vi "CONEX-PP-example.vi"(8 "error in (no error)":errorcluster, 9 "Input Value":string, 10 "Enum":T1(ring), 11 "VISA resource name":refnum<visa-resource-name>="COM6") -> (0 "error out read":errorcluster, 2 "Position":dbl)   [LabVIEW 2020]
doc: "This example performs a serial port write and a serial port read. The parameters set for the serial port must match the parameters of the connected instrument or device. The VISA Configure Serial Port VI sets the configuration parameters. The front panel displays the controls used to configure the basic parameters, such as baud rate, data bits, and parity. The VI passes the VISA resource name to other VIs that perform operations on that VISA resource. The VISA Write function sends a command to the serial device and the VISA Read function returns data based on the command. The VISA Close function then closes the reference to the serial device. It is important to close the reference; otherwise, further communication through that port might not be possible."
uses:
  Serial - Settings.ctl
panel:
  out "Velocity":dbl
  out "Acceleration":dbl
  out "error out write":errorcluster
  out "String 2":string
  in  "Serial Settings":T2={"baud rate"=115200, "data bits"=8, "parity"=enum."None", "stop bits"=10, "flow control"=0} {"flow control" items=["None"=0, "XON/XOFF"=1, "RTS/CTS"=2, "DTR/DSR"=4]; "stop bits" items=["1.0"=10, "1.5"=15, "2.0"=20]; "data bits" min=5 max=8 step=1; "baud rate" items=["75"=75, "110"=110, "134"=134, "150"=150, "300"=300, "600"=600, "1200"=1200, "1800"=1800, "2400"=2400, "4800"=4800, "7200"=7200, "9600"=9600, "14400"=14400, "19200"=19200, "28800"=28800, "38400"=38400, "56000"=56000, "57600"=57600, "115200"=115200, "128000"=128000, "230400"=230400]}
  out "bytes read":u32
  in  "delay before read (ms)":u32=500
  out "Response":string
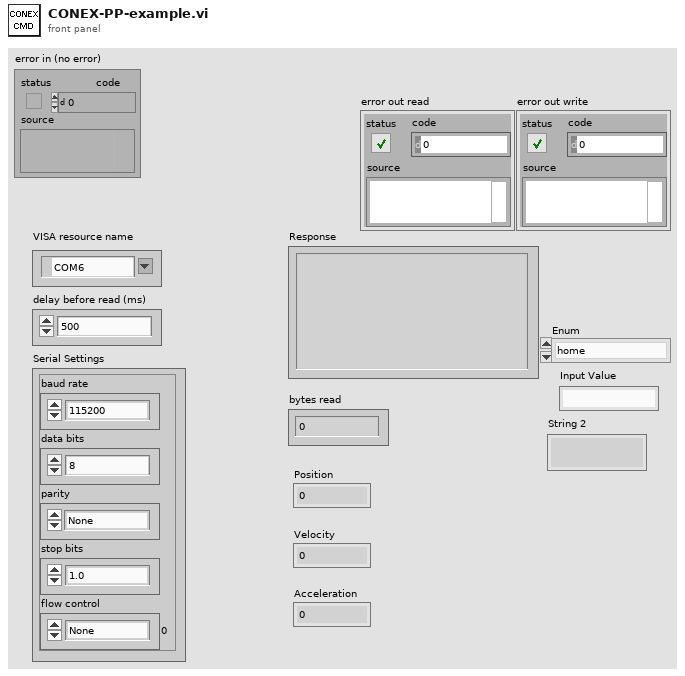
[diagram p1: front panel]
types:
  T1 = enum16{"home", "set position", "get position", "set velocity", "get velocity", "set acceleration", "get acceleration", "abort move", "get configuration", "reset controller", "custom command"}
  T2 = typedef "Serial - Settings.ctl" = cluster{"baud rate":u32, "data bits":u16, "parity":enum16{"None", "Odd", "Even", "Mark", "Space"}, "stop bits":u16, "flow control":u16}
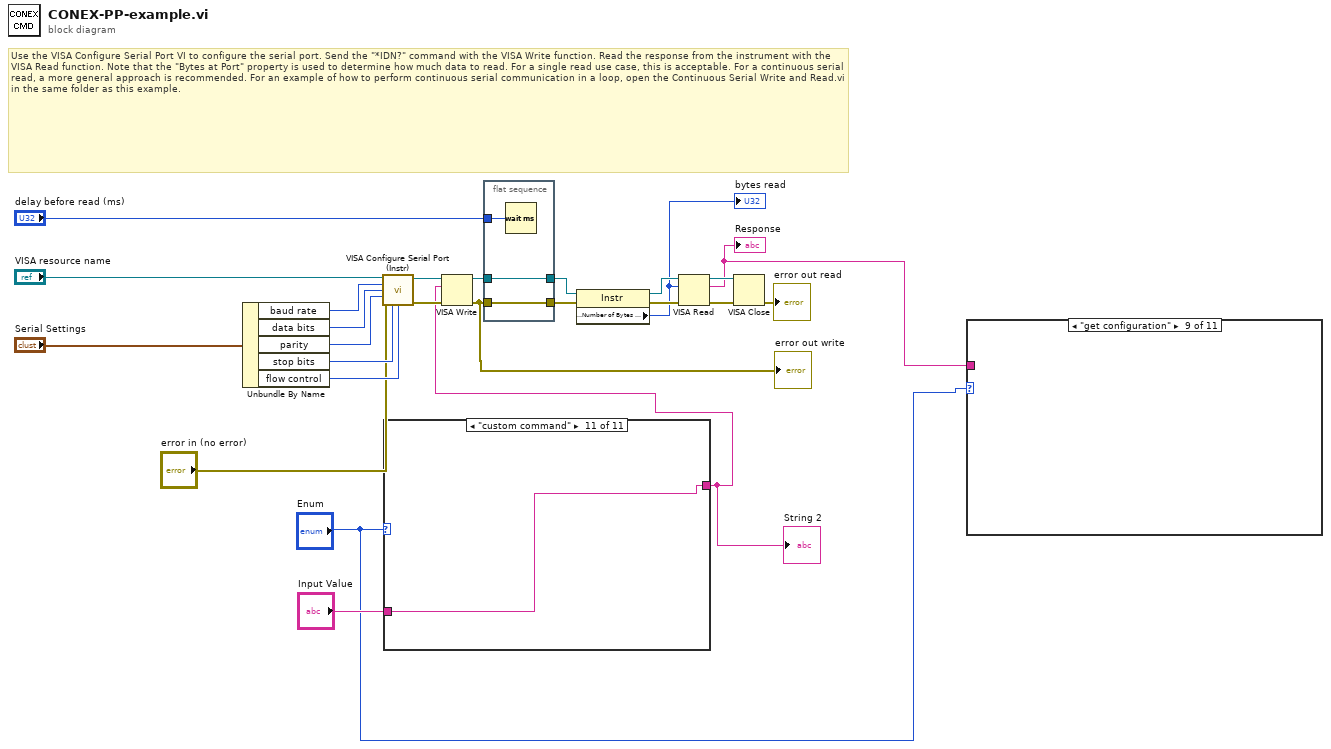
[diagram p0: block diagram]
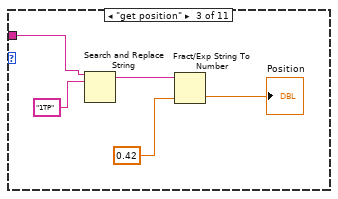
[diagram p4: hidden frame]
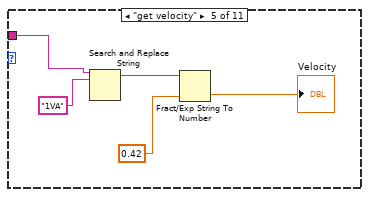
[diagram p6: hidden frame]
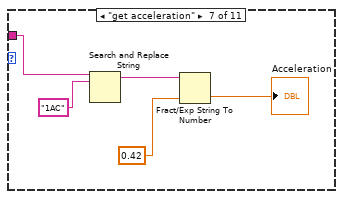
[diagram p8: hidden frame]
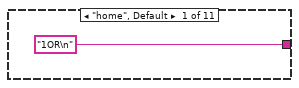
[diagram p12: hidden frame]
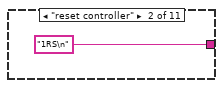
[diagram p13: hidden frame]
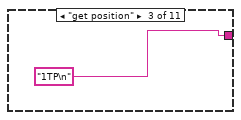
[diagram p14: hidden frame]
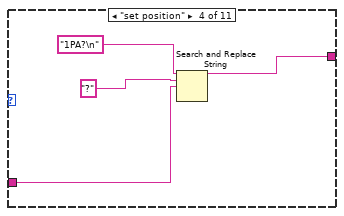
[diagram p15: hidden frame]
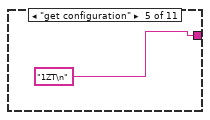
[diagram p16: hidden frame]
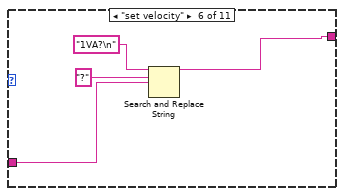
[diagram p17: hidden frame]
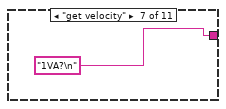
[diagram p18: hidden frame]
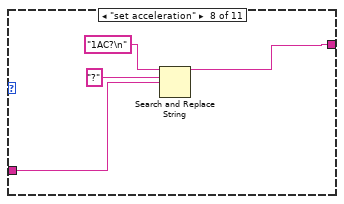
[diagram p19: hidden frame]
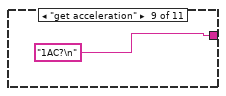
[diagram p20: hidden frame]
diagram:
  # "Use the VISA Configure Serial Port VI to configure the serial port. Send the \"*IDN?\" command with the VISA Write function. Read the response from the instrument with the VISA Read function. Note that the \"Bytes at Port\" property is used to determine how much data to read. For a single read use case, this is acceptable. For a continuous serial read, a more general approach is recommended. For an example of how to perform continuous serial communication in a loop, open the Continuous Serial Write and Read.vi in the same folder as this example."
  n1 = Unbundle By Name("Serial Settings") -> ("baud rate"=w12:u32, "data bits"=w11:u16, "parity"=w10:enum16{"None", "Odd", "Even", "Mark", "Space"}, "stop bits"=w9:u16, "flow control"=w8:u16)
  n2 = call "VISA Configure Serial Port (Instr).vi"("VISA resource name"="VISA resource name", "baud rate (9600)"=w12, "data bits (8)"=w11, "parity (0:none)"=w10, "error in (no error)"="error in (no error)", "stop bits (10: 1 bit)"=w9, "flow control (0:none)"=w8) -> ("VISA resource name out"=w23:refnum<visa-resource-name>, "error out"=w24:errorcluster)  [unwired: 7 in]
  n3 = case shown="\"custom command\"" "Enum" {
    tunnel: ["1OR\n" ("Command") "1RS\n" "1TP\n" w30 "1ZT\n" w34 "1VA?\n" w39 "1AC?\n" "1ST\n" w45] -> w6
    tunnel: "Input Value" -> [_ _ _ w29 _ w37 _ w40 _ _ w45]
    frame "home", Default {
    }
    frame "reset controller" {
    }
    frame "get position" {
    }
    frame "set position" {
      n4 = Search and Replace String(input string="1PA?\n", search string="?", replace string=w29) -> (result string=w30:string)  [unwired: 5 in, 3 out]
    }
    frame "get configuration" {
    }
    frame "set velocity" {
      n5 = Search and Replace String(input string="1VA?\n", search string="?", replace string=w37) -> (result string=w34:string)  [unwired: 5 in, 3 out]
    }
    frame "get velocity" {
    }
    frame "set acceleration" {
      n6 = Search and Replace String(input string="1AC?\n", search string="?", replace string=w40) -> (result string=w39:string)  [unwired: 5 in, 3 out]
    }
    frame "get acceleration" {
    }
    frame "abort move" {
    }
    frame "custom command" {
    }
  }
  "String 2" <- w6
  n7 = VISA Write(VISA resource name=w23, write buffer=w6, error in (no error)=w24) -> (VISA resource name out=w19:refnum<visa-resource-name>, error out=w4:errorcluster)  [unwired: 1 out]
  "error out write" <- w4
  n8 = flat-sequence {
    tunnel: w4 -> [w47]
    tunnel: [w47] -> w20
    tunnel: w19 -> [w46]
    tunnel: [w46] -> w18
    tunnel: "delay before read (ms)" -> [w48]
    frame #0 {
      n9 = Wait (ms)(milliseconds to wait=w48) -> ()  [unwired: 1 out]
    }
  }
  n10 = property class="Instr"(reference=w18, error in=w20) -> (reference out=w16:refnum<visa-resource-name>, error out=w15:errorcluster, "Serial Settings:Number of Bytes at Serial Port"=w14:u32)
  "bytes read" <- w14
  n11 = VISA Read(VISA resource name=w16, byte count=w14, error in (no error)=w15) -> (VISA resource name out=w21:refnum<visa-resource-name>, read buffer=w2:string, error out=w22:errorcluster)  [unwired: 1 out]
  "Response" <- w2
  n12 = VISA Close(VISA resource name=w21, error in (no error)=w22) -> (error out=→"error out read":errorcluster)
  n13 = case shown="\"get configuration\"" "Enum" {
    tunnel: w2 -> [_ _ w53 _ w55 _ w60 _ _ _ _]
    frame "home", Default {
    }
    frame "set position" {
    }
    frame "get position" {
      n14 = Search and Replace String(input string=w53, search string="1TP") -> (result string=w52:string)  [unwired: 6 in, 3 out]
      n15 = Fract/Exp String To Number(string=w52, default (0 dbl)=0.42) -> (number=→"Position":dbl)  [unwired: 2 in, 1 out]
    }
    frame "set velocity" {
    }
    frame "get velocity" {
      n16 = Search and Replace String(input string=w55, search string="1VA") -> (result string=w58:string)  [unwired: 6 in, 3 out]
      n17 = Fract/Exp String To Number(string=w58, default (0 dbl)=0.42) -> (number=→"Velocity":dbl)  [unwired: 2 in, 1 out]
    }
    frame "set acceleration" {
    }
    frame "get acceleration" {
      n18 = Search and Replace String(input string=w60, search string="1AC") -> (result string=w63:string)  [unwired: 6 in, 3 out]
      n19 = Fract/Exp String To Number(string=w63, default (0 dbl)=0.42) -> (number=→"Acceleration":dbl)  [unwired: 2 in, 1 out]
    }
    frame "abort move" {
    }
    frame "get configuration" {
    }
    frame "reset controller" {
    }
    frame "custom command" {
    }
  }
